vi "f_ss1.vi"(4 "index in":i32, 5 "lower lim":i16, 6 "Y":i16[](array[numeric]), 7 "upper lim":i16, 8 "Boolean":bool caption="поиск") -> (0 "eof":bool, 1 "index out":i32, 3 "found":bool)   [LabVIEW 2010]
panel:
  # "on - подъёма\noff - спада"
  # "Если первым идет подъём\nпри поиске спада (спад при\nпоиске подъёма)\nиндексы на входе и выходе\nсовпадают"
  # "Просто конец массива"
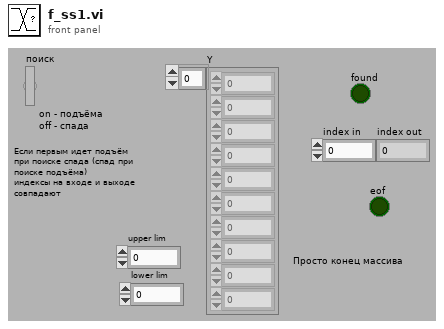
[diagram p1: front panel]
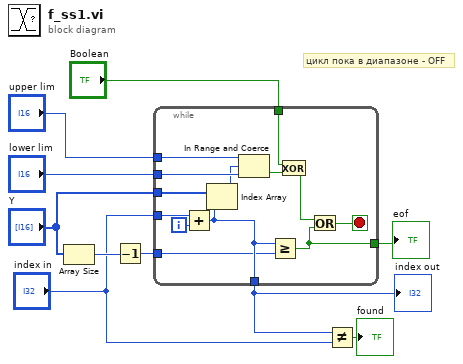
[diagram p0: block diagram]
diagram:
  # "цикл пока в диапазоне - OFF"
  n1 = Array Size(array="Y") -> (size(s)=w6:i32)
  n2 = Decrement(x=w6) -> (x-1=w5:i32)
  n3 = while "While not in range" {
    tunnel: "upper lim" -> [w23]
    tunnel: "lower lim" -> [w22]
    tunnel: "index in" -> [w20]
    tunnel: "Y" -> [w19]
    tunnel: [w15] -> w3
    tunnel: "Boolean" -> [w16]
    tunnel: w5 -> [w14]
    tunnel: [w11] -> w4
    i -> [w21]
    stop <- w12 stop-if-true
    n4 = Add(x=w20, y=w21) -> (x+y=w15:i32)
    n5 = Index Array(array=w19, index=w15) -> (element=w18:i16)
    n6 = In Range and Coerce(upper limit=w23, x=w18, lower limit=w22) -> (In Range?=w17:bool)  [unwired: 1 out]
    n7 = Greater Or Equal?(x=w15, y=w14) -> (x >= y?=w11:bool)
    n8 = Exclusive Or(1:w17, 2:w16) -> (0:w13:bool)
    n9 = Or(x=w13, y=w11) -> (x .or. y?=w12:bool)
  }
  "index out" <- w3
  "eof" <- w4
  n10 = Not Equal?(x=w3, y="index in") -> (x != y?=→"found":bool)
